vi "Random_Scale_Shift_Generator.vi"(10 "Shift":sgl, 11 "Scale":sgl) -> (1 "Shift  (W)":sgl, 2 "Shift (H)":sgl, 3 "Scale":sgl)   [LabVIEW 2020]
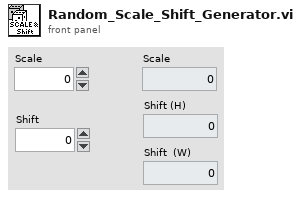
[diagram p1: front panel]
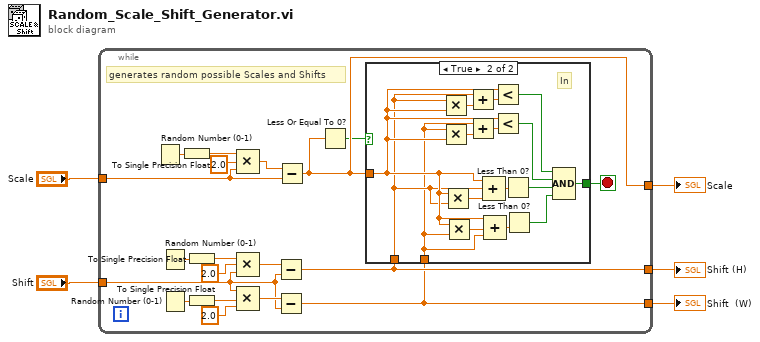
[diagram p0: block diagram]
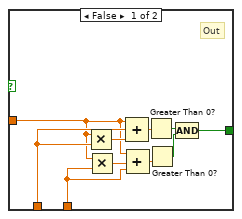
[diagram p2: hidden frame]
diagram:
  n1 = while {
    tunnel: "Scale" -> [w24]
    tunnel: [w7] -> w5
    tunnel: "Shift" -> [w9]
    tunnel: [w14] -> w3
    tunnel: [w8] -> w4
    stop <- w23 stop-if-true
    # "generates random possible Scales and Shifts"
    n2 = Random Number (0-1)() -> (number: 0 to 1=w18:dbl)
    n3 = Random Number (0-1)() -> (number: 0 to 1=w21:dbl)
    n4 = Random Number (0-1)() -> (number: 0 to 1=w11:dbl)
    n5 = To Single Precision Float(number=w18) -> (single precision float=w17:sgl)
    n6 = To Single Precision Float(number=w21) -> (single precision float=w20:sgl)
    n7 = To Single Precision Float(number=w11) -> (single precision float=w12:sgl)
    n8 = Compound Arithmetic op=MULTIPLY(w17, sgl 2.0 ("value"), w24) -> (w15:sgl)
    n9 = Compound Arithmetic op=MULTIPLY(w20, sgl 2.0 ("Shift"), w9) -> (w22:sgl)
    n10 = Compound Arithmetic op=MULTIPLY(w9, w12, sgl 2.0 ("Shift")) -> (w10:sgl)
    n11 = Subtract(x=w22, y=w9) -> (x-y=w14:sgl)
    n12 = Subtract(x=w10, y=w9) -> (x-y=w8:sgl)
    n13 = Subtract(x=w15, y=w24) -> (x-y=w7:sgl)
    n14 = Less Or Equal To 0?(x=w7) -> (x <= 0?=w6:bool)
    n15 = case shown="True" w6 {
      tunnel: w7 -> [w27 w38]
      tunnel: [w25 w37] -> w23
      tunnel: w14 -> [w28 w36]
      tunnel: w8 -> [w26 w35]
      frame False {
        # "Out"
        n16 = Multiply(x=w27, y=w28) -> (x*y=w32:sgl)
        n17 = Multiply(x=w27, y=w26) -> (x*y=w29:sgl)
        n18 = Compound Arithmetic op=ADD(w27, w28, w32) -> (w31:sgl)
        n19 = Compound Arithmetic op=ADD(w27, w29, w26) -> (w30:sgl)
        n20 = Greater Than 0?(x=w31) -> (x > 0?=w33:bool)
        n21 = Greater Than 0?(x=w30) -> (x > 0?=w34:bool)
        n22 = Compound Arithmetic op=AND(w33, w34) -> (w25:bool)
      }
      frame True {
        # "In"
        n23 = Multiply(x=w36, y=w38) -> (x*y=w50:sgl)
        n24 = Multiply(x=w35, y=w38) -> (x*y=w46:sgl)
        n25 = Multiply(x=w38, y=w36) -> (x*y=w44:sgl)
        n26 = Multiply(x=w38, y=w35) -> (x*y=w40:sgl)
        n27 = Add(x=w36, y=w50) -> (x+y=w49:sgl)
        n28 = Add(x=w35, y=w46) -> (x+y=w47:sgl)
        n29 = Compound Arithmetic op=ADD(w38, w36, w44) -> (w43:sgl)
        n30 = Compound Arithmetic op=ADD(w38, w40, w35) -> (w41:sgl)
        n31 = Less?(x=w38, y=w49) -> (x < y?=w48:bool)
        n32 = Less?(x=w38, y=w47) -> (x < y?=w45:bool)
        n33 = Less Than 0?(x=w43) -> (x < 0?=w42:bool)
        n34 = Less Than 0?(x=w41) -> (x < 0?=w39:bool)
        n35 = Compound Arithmetic op=AND(w48, w45, w42, w39) -> (w37:bool)
      }
    }
  }
  "Scale" <- w5
  "Shift  (W)" <- w4
  "Shift (H)" <- w3
